vi "Read Waveform.vi"(8 "error in (no error)":errorcluster, 11 "Tektronix TDS 200 1000 2000 in":refnum<class "Tektronix TDS 200 1000 2000.lvclass">) -> (0 "error out":errorcluster, 2 "Waveform Data":waveform(dbl)[](graph), 3 "Tektronix TDS 200 1000 2000 out":refnum<class "Tektronix TDS 200 1000 2000.lvclass">)   [LabVIEW 2020, in "Tektronix TDS 200 1000 2000.lvclass"]
uses:
  Tektronix TDS 200 1000 2000.lvclass
  C:/Sandbox/Git_Sandbox/WiSpry Test Framework source code (LV20)/WiSpry Test Framework/Instruments/Instrument.lvclass
  Instrument.lvclass/Instrument.ctl
  <instrlib>/Tektronix TDS 200 1000 2000 Series/Public/Data/Read (Multiple Waveforms).vi
  Instrument.lvclass
  <instrlib>/Tektronix TDS 200 1000 2000 Series/Tektronix TDS 200 1000 2000 Series.lvlib
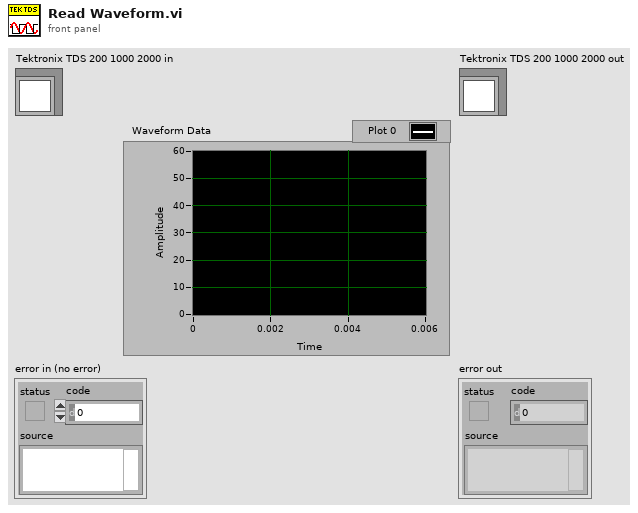
[diagram p1: front panel]
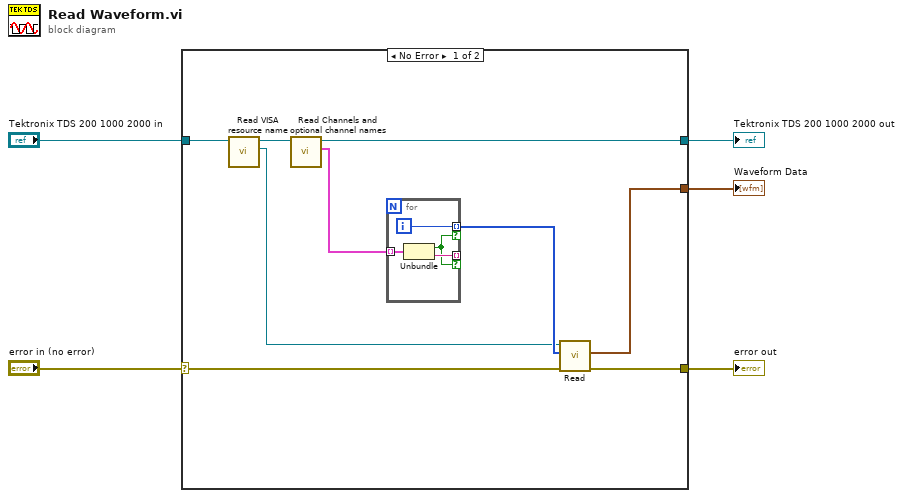
[diagram p0: block diagram]
diagram:
  n1 = case shown="No Error" "error in (no error)" {
    selector: "error in (no error)" -> [w7 w20]
    tunnel: [w10 w20] -> w4
    tunnel: [w11 w19] -> w3
    tunnel: "Tektronix TDS 200 1000 2000 in" -> [w14 w19]
    tunnel: [w9 _] -> w1
    frame No Error {
      n2 = call "Read VISA resource name.vi"("Instrument in"=w14) -> ("VISA resource name"=w6:refnum<visa-resource-name>, "Instrument out"=w13:refnum<class "Tektronix TDS 200 1000 2000.lvclass">)  [unwired: 9 in]
      n3 = call-dynamic "Read Channels and optional channel names.vi"("Oscilloscope in"=w13) -> ("Channels and optional channel names"=w12:cluster{"Enabled":bool, "Channel name":string}[], "Oscilloscope out"=w11:refnum<class "Tektronix TDS 200 1000 2000.lvclass">)  [unwired: 9 in]
      n4 = for {
        tunnel: w12 -> [w17] mode=indexing
        tunnel: [w18] -> w8 mode=indexing if=w15
        tunnel: [w16] -> _ mode=indexing if=w15
        i -> [w18]
        n5 = Unbundle(w17) -> ("Enabled"=w15:bool, "Channel name"=w16:string)
      }
      n6 = call-poly <instrlib>:"Read.vi"("error in (no error)"=w7, "Channels"=w8, "VISA resource name"=w6) -> ("error out"=w10:errorcluster, "Waveform Data"=w9:waveform(dbl)[])  [unwired: 6 in, 1 out]
    }
    frame Error {
    }
  }
  "error out" <- w4
  "Tektronix TDS 200 1000 2000 out" <- w3
  "Waveform Data" <- w1
